vi "PH_Beckhoff.set Connectivity GUI Object.vi"(1 "GUI Ref Connection":refnum<vi>, 3 "Connection":T1, 5 "error in":errorcluster) -> (19 "error out":errorcluster)   [LabVIEW 2014, in "PH_Beckhoff.lvlib"]
uses:
  PH_Beckhoff.lvlib
  PH_Beckhoff.Connectivity.ctl
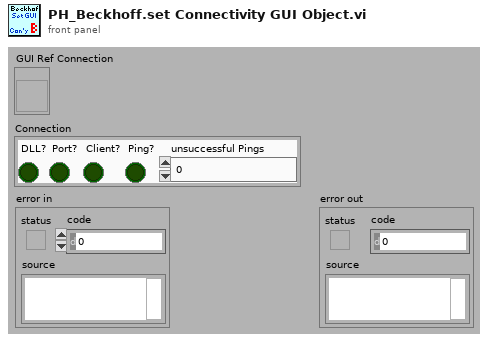
[diagram p1: front panel]
types:
  T1 = typedef "PH_Beckhoff.lvlib/PH_Beckhoff.Connectivity.ctl" = cluster{"DLL?":bool, "Port?":bool, "Client?":bool, "Ping?":bool, "unsuccessful Pings":u32}
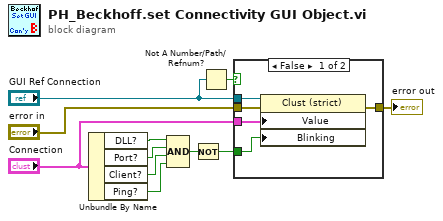
[diagram p0: block diagram]
diagram:
  n1 = Unbundle By Name("Connection") -> ("DLL?"=w2:bool, "Port?"=w7:bool, "Client?"=w6:bool, "Ping?"=w5:bool)
  n2 = Compound Arithmetic op=AND(w2, w7, w6, w5) -> (w4:bool)
  n3 = Not(x=w4) -> (.not. x?=w3:bool)
  n4 = Not A Number/Path/Refnum?(number/path/refnum="GUI Ref Connection") -> (NaN/Path/Refnum?=w9:bool)
  n5 = case shown="False" w9 {
    tunnel: "Connection" -> [w16 _]
    tunnel: [w15 w17] -> w11
    tunnel: "error in" -> [w14 w17]
    tunnel: "GUI Ref Connection" -> [w13 _]
    tunnel: w3 -> [w12 _]
    frame False {
      n6 = property class="Clust (strict)"(reference=w13, error in=w14, "Value"=w16, "Blinking"=w12) -> (error out=w15:errorcluster)  [unwired: 1 out]
    }
    frame True {
    }
  }
  "error out" <- w11
